vi "Diesel Engine Factory_Create.vi"(0 "reference in":refnum<class "Diesel Engine Factory.lvclass">, 11 "Error In":errorcluster) -> (4 "reference out":refnum<class "Diesel Engine Factory.lvclass">, 15 "Error Out":errorcluster)   [LabVIEW 2024, in "Diesel Engine Factory.lvclass"]
uses:
  Diesel Engine Factory.lvclass
  C:/Users/burakkorkmaz/Desktop/Leveling/labview-desing-patterns/Abstract Factory Pattern/EngineFactory/EngineFactory.lvclass
  Diesel Engine Factory.lvclass/Diesel Engine Factory.ctl
  EngineFactory/EngineFactory.lvclass
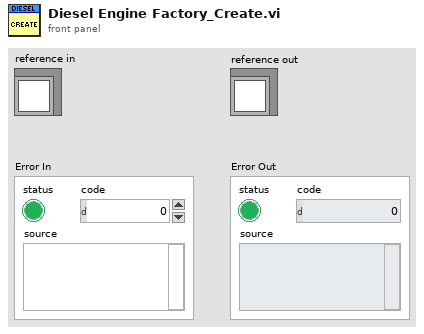
[diagram p1: front panel]
types:
  T1 = typedef "Diesel Engine Factory.lvclass/ObjectAttributes.ctl" = cluster{"None":bool}
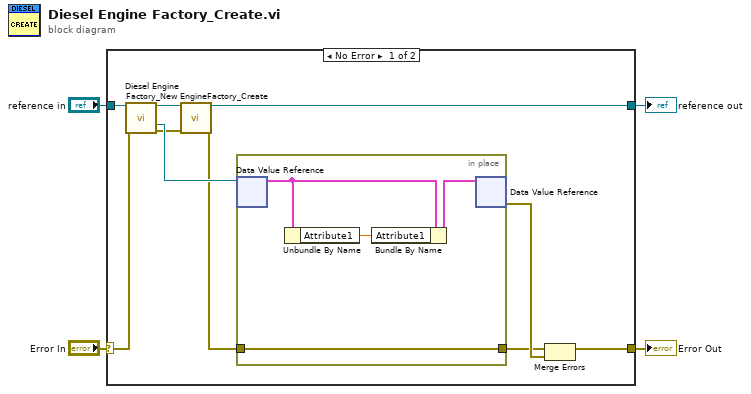
[diagram p0: block diagram]
diagram:
  n1 = case shown="No Error" "Error In" {
    selector: "Error In" -> [w10 w20]
    tunnel: [w8 w20] -> w3
    tunnel: "reference in" -> [w12 w19]
    tunnel: [w7 w19] -> w1
    frame No Error {
      n2 = call "Diesel Engine Factory_New.vi"("reference in"=w12, "Error In"=w10) -> ("reference out"=w13:refnum<class "Diesel Engine Factory.lvclass">, "DVRRefOut"=w14:refnum<data-value>, "Error Out"=w11:errorcluster)  [unwired: 10 in, 1 out]
      n3 = call "EngineFactory_Create.vi"("reference in"=w13, "Error In"=w11) -> ("reference out"=w7:refnum<class "Diesel Engine Factory.lvclass">, "Error Out"=w6:errorcluster)  [unwired: 12 in]
      n4 = in-place {
        in-place-border: w6 -> [w15]
        in-place-border: [w15] -> w5
        n5 = in-place-dvr #1(w14) -> (w17:T1)  [unwired: 1 out]
        n6 = Unbundle By Name(w17) -> ("Attribute1"=w16:dbl)
        n7 = Bundle By Name(cluster=w17, "Attribute1"=w16) -> (w18:T1)
        n8 = in-place-dvr #1(w18) -> (w9:errorcluster)  [unwired: 1 out]
      }
      n9 = Merge Errors(w5, w9) -> (w8:errorcluster)
    }
    frame Error {
    }
  }
  "Error Out" <- w3
  "reference out" <- w1
